vi "svx_Oct_Waterfall Facade.vi"(0 "Data In":T2={"z0"=0.0, "dz"=1.0, "Plots"=[]} {"Plots"."Y" format="%.2f"; "Plots"."X" format="%.2f"}, 2 "Display State In":T5={"X Scale Width %"=50.0, "Y Scale Height %"=50.0, "X-Axis Range"={"Minimum"=0.0, "Maximum"=10.0}, "Y-Axis Range"={"Minimum"=0.0, "Maximum"=10.0}, "Z-Axis Range"={"Minimum"=0.0, "Maximum"=10.0}, "Plot Color"=0, "Frame Color"=61212, "Background Color"=16252785, "Initial AutoScale Y"=TRUE, "AutoScale X"=2, "AutoScale Y"=2, "AutoScale Z"=2, "Plot Transparency"=FALSE, "X-Axis Name"="Frequency", "Y-Axis Name"="Amplitude", "Z-Axis Name"="", "X-Axis Scaling Factor"={"Offset"=0.0, "Multiplier"=1.0}, "Y-Axis Scaling Factor"={"Offset"=0.0, "Multiplier"=1.0}, "Z-Axis Scaling Factor"={"Offset"=0.0, "Multiplier"=1.0}, "X-Scale Visible"=TRUE, "Y-Scale Visible"=TRUE, "Z-Scale Visible"=TRUE, "X-Scale Label Visible"=TRUE, "Y-Scale Label Visible"=TRUE, "Z-Scale Label Visible"=TRUE, "X-Axis Range Scaled"={"Minimum"=0.0, "Maximum"=10.0}, "Y-Axis Range Scaled"={"Minimum"=0.0, "Maximum"=10.0}, "Z-Axis Range Scaled"={"Minimum"=0.0, "Maximum"=10.0}, "Rev Z Order"=FALSE, "X-Scale Format Str"="%#.4g", "Y-Scale Format Str"="%#.4g", "Z-Scale Format Str"="%#.4g", "Decor color"=12369084, "Scale Range Change"=refnum, "out of state queue"=refnum, "property nodes"=refnum}, 3 "Container State":T6) -> (6 "Data Out":T2={"z0"=0.0, "dz"=1.0, "Plots"=[]} {"Plots"."Y" format="%.2f"; "Plots"."X" format="%.2f"}, 7 "Display State Out":T5={"X Scale Width %"=50.0, "Y Scale Height %"=50.0, "X-Axis Range"={"Minimum"=0.0, "Maximum"=10.0}, "Y-Axis Range"={"Minimum"=0.0, "Maximum"=10.0}, "Z-Axis Range"={"Minimum"=0.0, "Maximum"=10.0}, "Plot Color"=0, "Frame Color"=61212, "Background Color"=16252785, "Initial AutoScale Y"=TRUE, "AutoScale X"=2, "AutoScale Y"=2, "AutoScale Z"=2, "Plot Transparency"=FALSE, "X-Axis Name"="Frequency", "Y-Axis Name"="Amplitude", "Z-Axis Name"="", "X-Axis Scaling Factor"={"Offset"=0.0, "Multiplier"=1.0}, "Y-Axis Scaling Factor"={"Offset"=0.0, "Multiplier"=1.0}, "Z-Axis Scaling Factor"={"Offset"=0.0, "Multiplier"=1.0}, "X-Scale Visible"=TRUE, "Y-Scale Visible"=TRUE, "Z-Scale Visible"=TRUE, "X-Scale Label Visible"=TRUE, "Y-Scale Label Visible"=TRUE, "Z-Scale Label Visible"=TRUE, "X-Axis Range Scaled"={"Minimum"=0.0, "Maximum"=10.0}, "Y-Axis Range Scaled"={"Minimum"=0.0, "Maximum"=10.0}, "Z-Axis Range Scaled"={"Minimum"=0.0, "Maximum"=10.0}, "Rev Z Order"=FALSE, "X-Scale Format Str"="%#.4g", "Y-Scale Format Str"="%#.4g", "Z-Scale Format Str"="%#.4g", "Decor color"=12369084, "Scale Range Change"=refnum, "out of state queue"=refnum, "property nodes"=refnum}, 8 "Action":T4)   [LabVIEW 2017, in "SVX Octave Waterfall Graph.xctl"]
uses:
  <vilib>/addons/_XControls/Octave Waterfall Graph/SVX Octave Waterfall Graph.xctl
  <vilib>/addons/_XControls/Octave Waterfall Graph/subVIs/svx_Oct_Waterfall Data.ctl
  <vilib>/_xctls/Container State.ctl
  <vilib>/addons/_XControls/Octave Waterfall Graph/subVIs/svx_Oct_Waterfall State.ctl
  <vilib>/_xctls/Action.ctl
  <vilib>/Utility/miscctls.llb/LVPoint32TypeDef.ctl
  <vilib>/addons/_XControls/Octave Waterfall Graph/subVIs/svx_Oct_Waterfall Execution Tasks.ctl
  <vilib>/Utility/cursorutil.llb/Set Cursor (Icon Pict).vi
  <vilib>/_xctls/XControlSupport.lvlib
panel:
  out "Coords":T1
  out "# Plots Updated":i32
  out "Dec/Cropped":T2={"z0"=0.0, "dz"=1.0, "Plots"=[]} {"Plots"."Y" format="%.2f"; "Plots"."X" format="%.2f"}
  out "Main Graph":T3(graph)
  out "Z Scale Graph":cluster{"f0":dbl, "df":dbl, "magnitude":dbl[]}[](graph)
  out "XY Scale Graph":cluster{"f0":dbl, "df":dbl, "magnitude":dbl[]}[](graph)
  out "background":bool
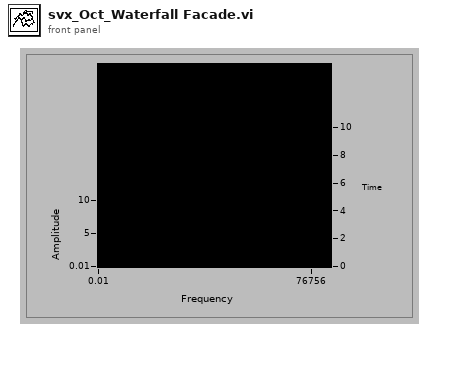
[diagram p1: front panel]
types:
  T1 = typedef "LVPoint32TypeDef.ctl" = cluster{"Horizontal":i32, "Vertical":i32}
  T2 = typedef "SVX Octave Waterfall Graph.xctl/svx_Oct_Waterfall Data.ctl" = cluster{"z0":dbl, "dz":dbl, "Plots":cluster{"X":dbl[], "Y":dbl[]}[]}
  T3 = cluster{"nominal frequencies [Hz]":dbl[], "band power [dB EU]":dbl[]}[]
  T4 = typedef "XControlSupport.lvlib/Action.ctl" = cluster{"Data Changed?":bool, "State Changed?":bool, "Action Name":string}
  T5 = typedef "SVX Octave Waterfall Graph.xctl/svx_Oct_Waterfall State.ctl" = cluster{"X Scale Width %":dbl, "Y Scale Height %":dbl, "X-Axis Range":cluster{"Minimum":dbl, "Maximum":dbl}, "Y-Axis Range":cluster{"Minimum":dbl, "Maximum":dbl}, "Z-Axis Range":cluster{"Minimum":dbl, "Maximum":dbl}, "Plot Color":u32, "Frame Color":u32, "Background Color":u32, "Initial AutoScale Y":bool, "AutoScale X":u8, "AutoScale Y":u8, "AutoScale Z":u8, "Plot Transparency":bool, "X-Axis Name":string, "Y-Axis Name":string, "Z-Axis Name":string, "X-Axis Scaling Factor":cluster{"Offset":dbl, "Multiplier":dbl}, "Y-Axis Scaling Factor":cluster{"Offset":dbl, "Multiplier":dbl}, "Z-Axis Scaling Factor":cluster{"Offset":dbl, "Multiplier":dbl}, "X-Scale Visible":bool, "Y-Scale Visible":bool, "Z-Scale Visible":bool, "X-Scale Label Visible":bool, "Y-Scale Label Visible":bool, "Z-Scale Label Visible":bool, "X-Axis Range Scaled":cluster{"Minimum":dbl, "Maximum":dbl}, "Y-Axis Range Scaled":cluster{"Minimum":dbl, "Maximum":dbl}, "Z-Axis Range Scaled":cluster{"Minimum":dbl, "Maximum":dbl}, "Rev Z Order":bool, "X-Scale Format Str":string, "Y-Scale Format Str":string, "Z-Scale Format Str":string, "Decor color":u32, "Scale Range Change":refnum<user-event>, "out of state queue":refnum<queue>, "property nodes":refnum<queue>}
  T6 = typedef "XControlSupport.lvlib/Container State.ctl" = cluster{"Indicator?":bool, "Run Mode?":bool, " Refnum":refnum<vi>}
  T7 = cluster{"Grabbing?":bool, "Coords":T1, "Time":u32}
  T8 = typedef "SVX Octave Waterfall Graph.xctl/svx_Oct_Waterfall Execution Tasks.ctl" = enum16{"[Data] Default", "[Data] Update Graph", "[Pane] Calculate Size from Coord Change", "[Pane] Calculate Size from Display State", "[Plot] Redraw Frame", "[Plot] Update Plot Color", "[Scale] Autoscale or Crop X, Y, Z", "[Scale] Resize Scales", "[Scale] Align Scale Labels", "[Plot] Initialize Plot", "[Scale] X Scale", "[Scale] Y Scale", "[Scale] Z Scale", "[Scale] Multiplier/Offset", "[Scale] Name", "[Scale] Visible", "[Scale] Label Visible", "[Scale] Format"}
  T9 = cluster{"use queue?":bool, "X-Axis Range":cluster{"Minimum":dbl, "Maximum":dbl}, "Y-Axis Range":cluster{"Minimum":dbl, "Maximum":dbl}, "Z-Axis Range":cluster{"Minimum":dbl, "Maximum":dbl}, "X-Axis Range Scaled":cluster{"Minimum":dbl, "Maximum":dbl}, "Y-Axis Range Scaled":cluster{"Minimum":dbl, "Maximum":dbl}, "Z-Axis Range Scaled":cluster{"Minimum":dbl, "Maximum":dbl}, "AutoScale X":u8, "AutoScale Y":u8, "AutoScale Z":u8, "background":refnum<vi>}
  T10 = cluster{"Scaled.Minimum":dbl, "Scaled.Maximum":dbl, "Kind":enum16{"X-Scale", "Y-Scale", "Z-Scale"}}
  T11 = cluster{"Range.Minimum":dbl, "Range.Maximum":dbl, "Kind":enum16{"X-Scale", "Y-Scale", "Z-Scale"}}
  T12 = typedef "LVRectTypeDef.ctl" = cluster{"Left":i16, "Top":i16, "Right":i16, "Bottom":i16}
  T13 = typedef "LVPositionTypeDef.ctl" = cluster{"Left":i32, "Top":i32}
  T14 = cluster{"Shift":bool, "Ctrl":bool, "Alt":bool, "Cmd":bool, "Opt":bool}
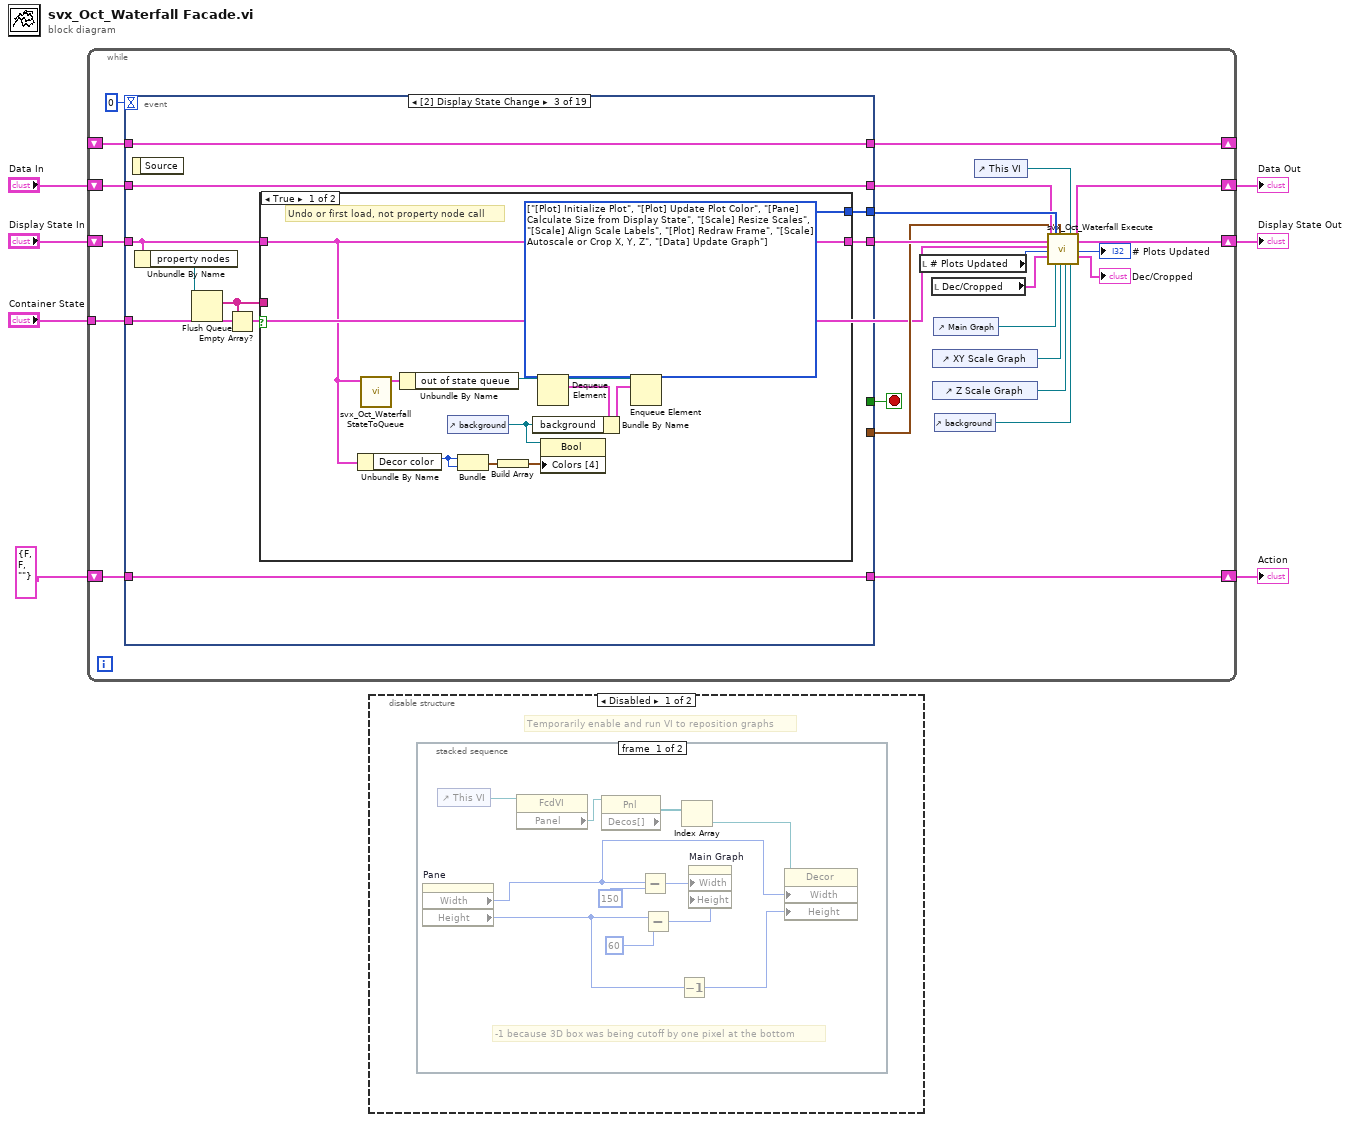
[diagram p0: block diagram]
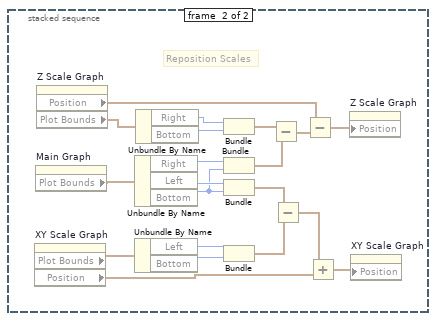
[diagram p2: hidden frame]
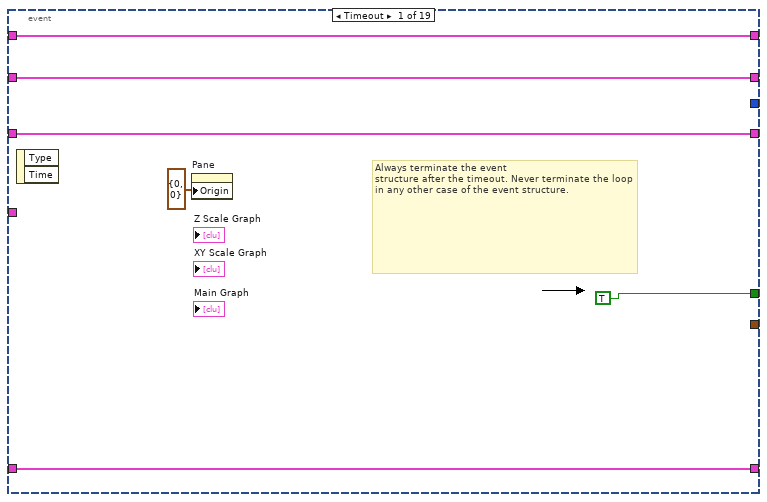
[diagram p4: hidden frame]
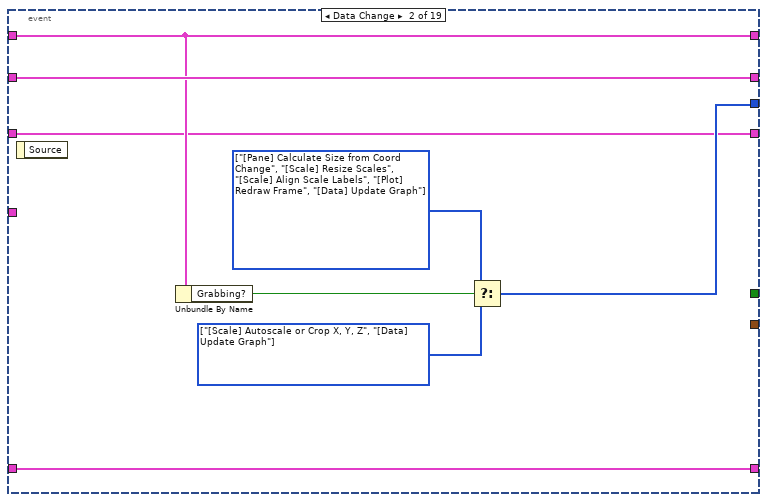
[diagram p5: hidden frame]
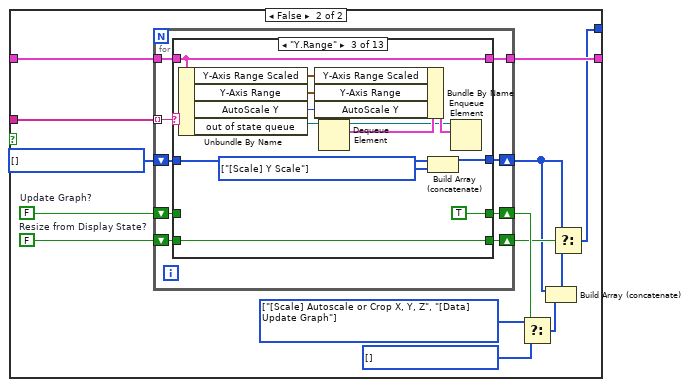
[diagram p6: hidden frame]
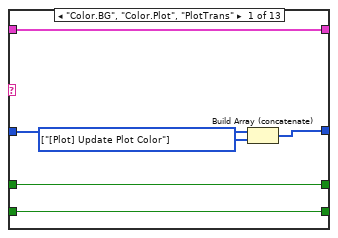
[diagram p7: hidden frame]
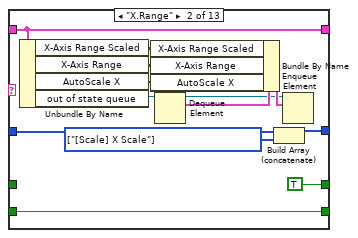
[diagram p8: hidden frame]
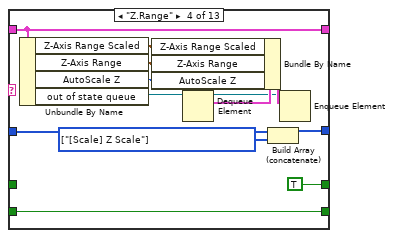
[diagram p9: hidden frame]
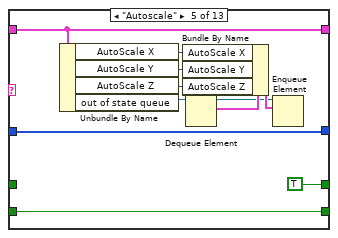
[diagram p10: hidden frame]
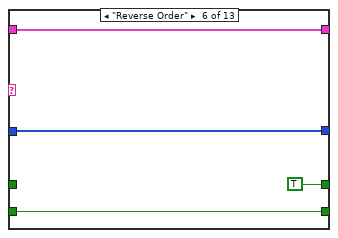
[diagram p11: hidden frame]
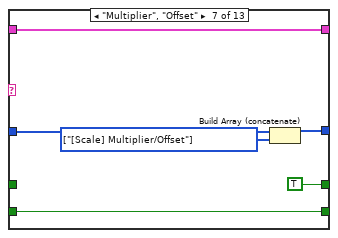
[diagram p12: hidden frame]
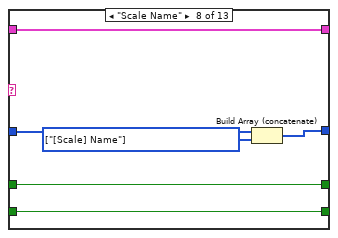
[diagram p13: hidden frame]
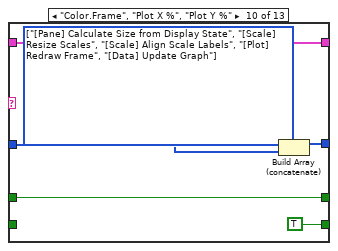
[diagram p15: hidden frame]
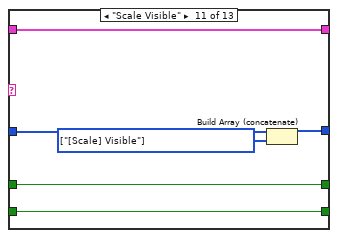
[diagram p16: hidden frame]
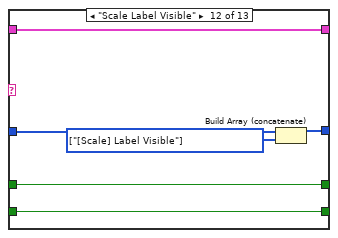
[diagram p17: hidden frame]
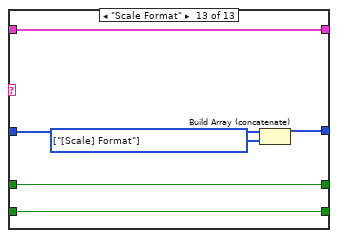
[diagram p18: hidden frame]
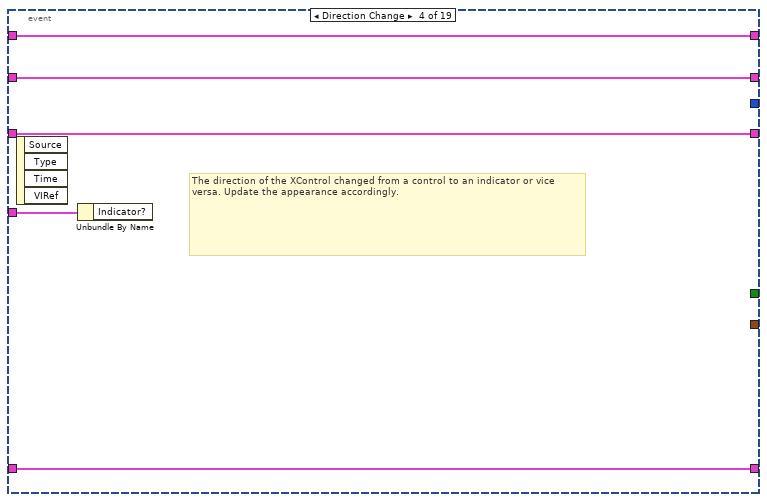
[diagram p19: hidden frame]
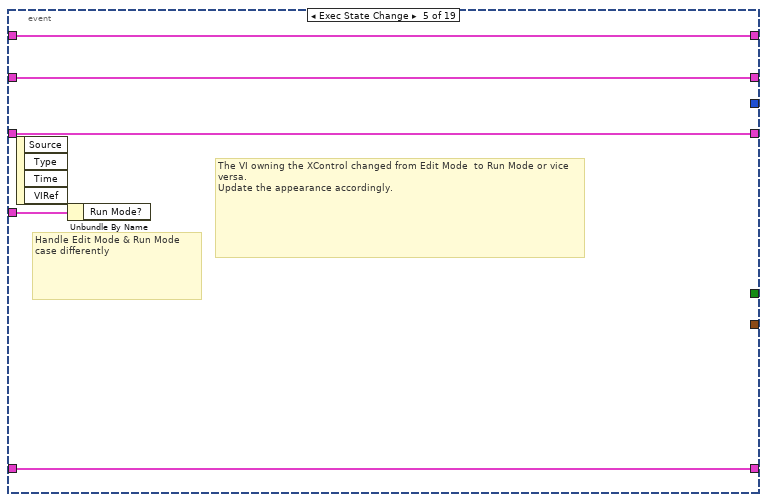
[diagram p20: hidden frame]
diagram:
  n1 = while {
    shift-right: [w12] -> w4
    shift-left: "Display State In" -> [w31]
    tunnel: "Container State" -> [w17]
    shift-right: [w20] -> w7
    shift-left: "Data In" -> [w28]
    shift-right: [w24] -> w2
    shift-left: T4 {"Data Changed?"=FALSE, "State Changed?"=FALSE, "Action Name"=""} ("Action") -> [w27]
    shift-right: [w25] -> _
    shift-left: _ -> [w26]
    stop <- w30 stop-if-true
    n2 = event shown="[2] Display State Change" {
      selector: _ -> [_ _ _ _ _ _ _ _ _ _ _ _ _ _ _ _ _ _ _]
      dyn-events: _ -> [_ _ _ _ _ _ _ _ _ _ _ _ _ _ _ _ _ _ _]
      timeout: 0 -> [_ _ _ _ _ _ _ _ _ _ _ _ _ _ _ _ _ _ _]
      tunnel: w31 -> [w32 w38 w51 w192 w197 w200 w227 w255 w290 w308 w315 w325 w385 w405 w447 w461 w479 w628 w654]
      tunnel: [w32 w38 w52 w192 w197 w199 w227 w255 w290 w308 w314 w325 w386 w405 w447 w461 w478 w628 w654] -> w22
      tunnel: [TRUE _ _ _ _ _ _ _ _ _ _ _ _ _ _ _ _ _ _] -> w30
      tunnel: w17 -> [_ _ _ w193 w198 w206 _ w254 w285 _ _ _ _ _ w448 w460 w474 _ _]
      tunnel: w28 -> [w36 w45 w53 w191 w196 w215 w230 w259 w289 w310 w321 w336 w399 w407 w454 w463 w475 w632 w655]
      tunnel: [w36 w45 w53 w191 w196 w215 w230 w259 w289 w310 w321 w336 w399 w407 w454 w463 w475 w631 w655] -> w21
      tunnel: [w33 w42 w47 w190 w195 w203 w226 w252 w283 w307 w312 w338 w400 w406 w455 w464 w476 w629 w648] -> w24
      tunnel: w27 -> [w33 w42 w47 w190 w195 w204 w226 w253 w284 w307 w313 w339 w401 w406 w455 w464 w477 w630 w648]
      tunnel: [w34 w44 w54 w189 w194 w214 w240 w262 w288 w309 w320 w341 w403 w409 w453 w462 w480 w635 w656] -> w25
      tunnel: w26 -> [w34 w44 w54 w189 w194 _ w239 w261 w287 w309 w320 w341 w403 w409 w453 w462 w480 w635 w656]
      tunnel: [_ _ _ _ _ _ w228 w256 _ _ _ _ _ _ _ _ _ _ _] -> w18
      tunnel: [_ w39 w46 _ _ _ w225 w251 w282 _ _ w328 w370 w404 _ _ w473 w627 _] -> w23
      event Timeout {
        # "Always terminate the event\nstructure after the timeout. Never terminate the loop in any other case of the event structure."
        n3 = event-data() -> ()  [unwired: 1 in, 2 out]
        n4 = property on="Pane" class="Pane"("Origin"=cluster{"Horizontal":i16, "Vertical":i16} {"Horizontal"=0, "Vertical"=0}) -> ()  [unwired: 2 in, 2 out]
      }
      event Data Change {
        w40 = T8[] [enum."[Scale] Autoscale or Crop X, Y, Z", enum."[Data] Update Graph"] items=["[Data] Default", "[Data] Update Graph", "[Pane] Calculate Size from Coord Change", "[Pane] Calculate Size from Display State", "[Plot] Redraw Frame", "[Plot] Update Plot Color", "[Scale] Autoscale or Crop X, Y, Z", "[Scale] Resize Scales", "[Scale] Align Scale Labels", "[Plot] Initialize Plot", "[Scale] X Scale", "[Scale] Y Scale", "[Scale] Z Scale", "[Scale] Multiplier/Offset", "[Scale] Name", "[Scale] Visible", "[Scale] Label Visible", "[Scale] Format"] ("element")
        w41 = T8[] [enum."[Pane] Calculate Size from Coord Change", enum."[Scale] Resize Scales", enum."[Scale] Align Scale Labels", enum."[Plot] Redraw Frame", enum."[Data] Update Graph"] items=["[Data] Default", "[Data] Update Graph", "[Pane] Calculate Size from Coord Change", "[Pane] Calculate Size from Display State", "[Plot] Redraw Frame", "[Plot] Update Plot Color", "[Scale] Autoscale or Crop X, Y, Z", "[Scale] Resize Scales", "[Scale] Align Scale Labels", "[Plot] Initialize Plot", "[Scale] X Scale", "[Scale] Y Scale", "[Scale] Z Scale", "[Scale] Multiplier/Offset", "[Scale] Name", "[Scale] Visible", "[Scale] Label Visible", "[Scale] Format"] ("element")
        n5 = event-data() -> ()  [unwired: 1 in, 1 out]
        n6 = Unbundle By Name(w44) -> ("Grabbing?"=w43:bool)
        n7 = Select(t=w41, s=w43, f=w40) -> (s? t:f=w39:T8[])
      }
      event Display State Change {
        n8 = event-data() -> ()  [unwired: 1 in, 1 out]
        n9 = Unbundle By Name(w51) -> ("property nodes"=w50:refnum<queue>)
        n10 = Flush Queue(queue=w50) -> (remaining elements=w48:string[])  [unwired: 1 in, 2 out]
        n11 = Empty Array?(array=w48) -> (empty?=w49:bool)
        n12 = case shown="True" w49 {
          tunnel: [w61 w79] -> w52
          tunnel: w51 -> [w61 w78]
          tunnel: [w60 w66] -> w46
          tunnel: w48 -> [_ w77]
          frame True {
            w60 = T8[] [enum."[Plot] Initialize Plot", enum."[Plot] Update Plot Color", enum."[Pane] Calculate Size from Display State", enum."[Scale] Resize Scales", enum."[Scale] Align Scale Labels", enum."[Plot] Redraw Frame", enum."[Scale] Autoscale or Crop X, Y, Z", enum."[Data] Update Graph"] items=["[Data] Default", "[Data] Update Graph", "[Pane] Calculate Size from Coord Change", "[Pane] Calculate Size from Display State", "[Plot] Redraw Frame", "[Plot] Update Plot Color", "[Scale] Autoscale or Crop X, Y, Z", "[Scale] Resize Scales", "[Scale] Align Scale Labels", "[Plot] Initialize Plot", "[Scale] X Scale", "[Scale] Y Scale", "[Scale] Z Scale", "[Scale] Multiplier/Offset", "[Scale] Name", "[Scale] Visible", "[Scale] Label Visible", "[Scale] Format"]
            # "Undo or first load, not property node call"
            n13 = Unbundle By Name(w61) -> ("Decor color"=w57:u32)
            n14 = call <vilib>:"svx_Oct_Waterfall StateToQueue.vi"("State In"=w61) -> ("State Out"=w65:T5)  [unwired: 10 in]
            n15 = Unbundle By Name(w65) -> ("out of state queue"=w62:refnum<queue>)
            n16 = control-ref of="background"() -> (w58:refnum<vi>)
            n17 = Bundle("Decor color"=w57, "Decor color"=w57) -> (w55:cluster{"Decor color":u32, "Decor color":u32})  [unwired: 1 in]
            n18 = Build Array(w55) -> (w56:cluster{"Decor color":u32, "Decor color":u32}[])
            n19 = Dequeue Element(queue=w62) -> (queue out=w59:refnum<queue>, element=w63:T9)  [unwired: 2 in, 2 out]
            n20 = Bundle By Name(cluster=w63, "background"=w58) -> (w64:T9)
            n21 = property on="Property Node" class="Bool"(reference=w58, "Colors [4]"=w56) -> ()  [unwired: 1 in, 2 out]
            n22 = Enqueue Element(queue=w59, element=w64) -> ()  [unwired: 2 in, 3 out]
          }
          frame False {
            w71 = T8[] [] items=["[Data] Default", "[Data] Update Graph", "[Pane] Calculate Size from Coord Change", "[Pane] Calculate Size from Display State", "[Plot] Redraw Frame", "[Plot] Update Plot Color", "[Scale] Autoscale or Crop X, Y, Z", "[Scale] Resize Scales", "[Scale] Align Scale Labels", "[Plot] Initialize Plot", "[Scale] X Scale", "[Scale] Y Scale", "[Scale] Z Scale", "[Scale] Multiplier/Offset", "[Scale] Name", "[Scale] Visible", "[Scale] Label Visible", "[Scale] Format"]
            w72 = T8[] [enum."[Scale] Autoscale or Crop X, Y, Z", enum."[Data] Update Graph"] items=["[Data] Default", "[Data] Update Graph", "[Pane] Calculate Size from Coord Change", "[Pane] Calculate Size from Display State", "[Plot] Redraw Frame", "[Plot] Update Plot Color", "[Scale] Autoscale or Crop X, Y, Z", "[Scale] Resize Scales", "[Scale] Align Scale Labels", "[Plot] Initialize Plot", "[Scale] X Scale", "[Scale] Y Scale", "[Scale] Z Scale", "[Scale] Multiplier/Offset", "[Scale] Name", "[Scale] Visible", "[Scale] Label Visible", "[Scale] Format"]
            w76 = T8[] [] items=["[Data] Default", "[Data] Update Graph", "[Pane] Calculate Size from Coord Change", "[Pane] Calculate Size from Display State", "[Plot] Redraw Frame", "[Plot] Update Plot Color", "[Scale] Autoscale or Crop X, Y, Z", "[Scale] Resize Scales", "[Scale] Align Scale Labels", "[Plot] Initialize Plot", "[Scale] X Scale", "[Scale] Y Scale", "[Scale] Z Scale", "[Scale] Multiplier/Offset", "[Scale] Name", "[Scale] Visible", "[Scale] Label Visible", "[Scale] Format"]
            w74 = FALSE  # Resize from Display State?
            w75 = FALSE  # Update Graph?
            n23 = for {
              tunnel: [w88] -> w79
              tunnel: w77 -> [w87] mode=indexing
              tunnel: w78 -> [w86]
              shift-right: [w84] -> w68
              shift-left: w76 -> [w85]
              shift-right: [w83] -> w73
              shift-left: w75 -> [w82]
              shift-right: [w80] -> w70
              shift-left: w74 -> [w81]
              n24 = case shown="\"Y.Range\"" w87 {
                tunnel: [w94 w96 w110 w122 w135 w148 w154 w160 w164 w170 w176 w182 w188] -> w88
                tunnel: w86 -> [w94 w96 w110 w122 w135 w148 w154 w160 w164 w170 w176 w182 w188]
                tunnel: w85 -> [w93 w104 w117 w130 w144 w147 w150 w158 w163 w167 w172 w179 w185]
                tunnel: [w91 w105 w118 w131 w144 w147 w151 w157 w163 w168 w173 w180 w186] -> w84
                tunnel: [w90 TRUE ("Update Graph?") TRUE ("Update Graph?") TRUE ("Update Graph?") TRUE ("Update Graph?") TRUE ("Update Graph?") TRUE ("Update Graph?") w156 w162 w169 w175 w178 w184] -> w83
                tunnel: w82 -> [w90 _ _ _ _ _ _ w156 w162 w169 w175 w178 w184]
                tunnel: w81 -> [w89 w95 w109 w121 w134 w145 w149 w155 w161 _ w171 w177 w183]
                tunnel: [w89 w95 w109 w121 w134 w145 w149 w155 w161 TRUE ("Resize from Display State?") w171 w177 w183] -> w80
                frame "Color.BG", "Color.Plot", "PlotTrans" {
                  w92 = T8[] [enum."[Plot] Update Plot Color"] items=["[Data] Default", "[Data] Update Graph", "[Pane] Calculate Size from Coord Change", "[Pane] Calculate Size from Display State", "[Plot] Redraw Frame", "[Plot] Update Plot Color", "[Scale] Autoscale or Crop X, Y, Z", "[Scale] Resize Scales", "[Scale] Align Scale Labels", "[Plot] Initialize Plot", "[Scale] X Scale", "[Scale] Y Scale", "[Scale] Z Scale", "[Scale] Multiplier/Offset", "[Scale] Name", "[Scale] Visible", "[Scale] Label Visible", "[Scale] Format"] ("element")
                  n25 = Build Array (concatenate)(w93, w92) -> (w91:T8[])
                }
                frame "X.Range" {
                  w106 = T8[] [enum."[Scale] X Scale"] items=["[Data] Default", "[Data] Update Graph", "[Pane] Calculate Size from Coord Change", "[Pane] Calculate Size from Display State", "[Plot] Redraw Frame", "[Plot] Update Plot Color", "[Scale] Autoscale or Crop X, Y, Z", "[Scale] Resize Scales", "[Scale] Align Scale Labels", "[Plot] Initialize Plot", "[Scale] X Scale", "[Scale] Y Scale", "[Scale] Z Scale", "[Scale] Multiplier/Offset", "[Scale] Name", "[Scale] Visible", "[Scale] Label Visible", "[Scale] Format"] ("element")
                  n26 = Unbundle By Name(w96) -> ("X-Axis Range Scaled"=w101:cluster{"Minimum":dbl, "Maximum":dbl}, "X-Axis Range"=w103:cluster{"Minimum":dbl, "Maximum":dbl}, "AutoScale X"=w102:u8, "out of state queue"=w97:refnum<queue>)
                  n27 = Dequeue Element(queue=w97) -> (queue out=w98:refnum<queue>, element=w99:T9)  [unwired: 2 in, 2 out]
                  n28 = Bundle By Name(cluster=w99, "X-Axis Range Scaled"=w101, "X-Axis Range"=w103, "AutoScale X"=w102) -> (w100:T9)
                  n29 = Build Array (concatenate)(w104, w106) -> (w105:T8[])
                  n30 = Enqueue Element(queue=w98, element=w100) -> ()  [unwired: 2 in, 3 out]
                }
                frame "Y.Range" {
                  w119 = T8[] [enum."[Scale] Y Scale"] items=["[Data] Default", "[Data] Update Graph", "[Pane] Calculate Size from Coord Change", "[Pane] Calculate Size from Display State", "[Plot] Redraw Frame", "[Plot] Update Plot Color", "[Scale] Autoscale or Crop X, Y, Z", "[Scale] Resize Scales", "[Scale] Align Scale Labels", "[Plot] Initialize Plot", "[Scale] X Scale", "[Scale] Y Scale", "[Scale] Z Scale", "[Scale] Multiplier/Offset", "[Scale] Name", "[Scale] Visible", "[Scale] Label Visible", "[Scale] Format"] ("element")
                  n31 = Unbundle By Name(w110) -> ("Y-Axis Range Scaled"=w108:cluster{"Minimum":dbl, "Maximum":dbl}, "Y-Axis Range"=w115:cluster{"Minimum":dbl, "Maximum":dbl}, "AutoScale Y"=w116:u8, "out of state queue"=w112:refnum<queue>)
                  n32 = Dequeue Element(queue=w112) -> (queue out=w111:refnum<queue>, element=w113:T9)  [unwired: 2 in, 2 out]
                  n33 = Bundle By Name(cluster=w113, "Y-Axis Range Scaled"=w108, "Y-Axis Range"=w115, "AutoScale Y"=w116) -> (w114:T9)
                  n34 = Build Array (concatenate)(w117, w119) -> (w118:T8[])
                  n35 = Enqueue Element(queue=w111, element=w114) -> ()  [unwired: 2 in, 3 out]
                }
                frame "Z.Range" {
                  w132 = T8[] [enum."[Scale] Z Scale"] items=["[Data] Default", "[Data] Update Graph", "[Pane] Calculate Size from Coord Change", "[Pane] Calculate Size from Display State", "[Plot] Redraw Frame", "[Plot] Update Plot Color", "[Scale] Autoscale or Crop X, Y, Z", "[Scale] Resize Scales", "[Scale] Align Scale Labels", "[Plot] Initialize Plot", "[Scale] X Scale", "[Scale] Y Scale", "[Scale] Z Scale", "[Scale] Multiplier/Offset", "[Scale] Name", "[Scale] Visible", "[Scale] Label Visible", "[Scale] Format"] ("element")
                  n36 = Unbundle By Name(w122) -> ("Z-Axis Range Scaled"=w126:cluster{"Minimum":dbl, "Maximum":dbl}, "Z-Axis Range"=w127:cluster{"Minimum":dbl, "Maximum":dbl}, "AutoScale Z"=w125:u8, "out of state queue"=w124:refnum<queue>)
                  n37 = Dequeue Element(queue=w124) -> (queue out=w123:refnum<queue>, element=w128:T9)  [unwired: 2 in, 2 out]
                  n38 = Bundle By Name(cluster=w128, "Z-Axis Range Scaled"=w126, "Z-Axis Range"=w127, "AutoScale Z"=w125) -> (w129:T9)
                  n39 = Build Array (concatenate)(w130, w132) -> (w131:T8[])
                  n40 = Enqueue Element(queue=w123, element=w129) -> ()  [unwired: 2 in, 3 out]
                }
                frame "Autoscale" {
                  n41 = Unbundle By Name(w135) -> ("AutoScale X"=w140:u8, "AutoScale Y"=w141:u8, "AutoScale Z"=w142:u8, "out of state queue"=w137:refnum<queue>)
                  n42 = Dequeue Element(queue=w137) -> (queue out=w136:refnum<queue>, element=w138:T9)  [unwired: 2 in, 2 out]
                  n43 = Bundle By Name(cluster=w138, "AutoScale X"=w140, "AutoScale Y"=w141, "AutoScale Z"=w142) -> (w139:T9)
                  n44 = Enqueue Element(queue=w136, element=w139) -> ()  [unwired: 2 in, 3 out]
                }
                frame "Reverse Order" {
                }
                frame "Multiplier", "Offset" {
                  w152 = T8[] [enum."[Scale] Multiplier/Offset"] items=["[Data] Default", "[Data] Update Graph", "[Pane] Calculate Size from Coord Change", "[Pane] Calculate Size from Display State", "[Plot] Redraw Frame", "[Plot] Update Plot Color", "[Scale] Autoscale or Crop X, Y, Z", "[Scale] Resize Scales", "[Scale] Align Scale Labels", "[Plot] Initialize Plot", "[Scale] X Scale", "[Scale] Y Scale", "[Scale] Z Scale", "[Scale] Multiplier/Offset", "[Scale] Name", "[Scale] Visible", "[Scale] Label Visible", "[Scale] Format"] ("element")
                  n45 = Build Array (concatenate)(w150, w152) -> (w151:T8[])
                }
                frame "Scale Name" {
                  w159 = T8[] [enum."[Scale] Name"] items=["[Data] Default", "[Data] Update Graph", "[Pane] Calculate Size from Coord Change", "[Pane] Calculate Size from Display State", "[Plot] Redraw Frame", "[Plot] Update Plot Color", "[Scale] Autoscale or Crop X, Y, Z", "[Scale] Resize Scales", "[Scale] Align Scale Labels", "[Plot] Initialize Plot", "[Scale] X Scale", "[Scale] Y Scale", "[Scale] Z Scale", "[Scale] Multiplier/Offset", "[Scale] Name", "[Scale] Visible", "[Scale] Label Visible", "[Scale] Format"] ("element")
                  n46 = Build Array (concatenate)(w158, w159) -> (w157:T8[])
                }
                frame Default {
                }
                frame "Color.Frame", "Plot X %", "Plot Y %" {
                  w166 = T8[] [enum."[Pane] Calculate Size from Display State", enum."[Scale] Resize Scales", enum."[Scale] Align Scale Labels", enum."[Plot] Redraw Frame", enum."[Data] Update Graph"] items=["[Data] Default", "[Data] Update Graph", "[Pane] Calculate Size from Coord Change", "[Pane] Calculate Size from Display State", "[Plot] Redraw Frame", "[Plot] Update Plot Color", "[Scale] Autoscale or Crop X, Y, Z", "[Scale] Resize Scales", "[Scale] Align Scale Labels", "[Plot] Initialize Plot", "[Scale] X Scale", "[Scale] Y Scale", "[Scale] Z Scale", "[Scale] Multiplier/Offset", "[Scale] Name", "[Scale] Visible", "[Scale] Label Visible", "[Scale] Format"]
                  n47 = Build Array (concatenate)(w167, w166) -> (w168:T8[])
                }
                frame "Scale Visible" {
                  w174 = T8[] [enum."[Scale] Visible"] items=["[Data] Default", "[Data] Update Graph", "[Pane] Calculate Size from Coord Change", "[Pane] Calculate Size from Display State", "[Plot] Redraw Frame", "[Plot] Update Plot Color", "[Scale] Autoscale or Crop X, Y, Z", "[Scale] Resize Scales", "[Scale] Align Scale Labels", "[Plot] Initialize Plot", "[Scale] X Scale", "[Scale] Y Scale", "[Scale] Z Scale", "[Scale] Multiplier/Offset", "[Scale] Name", "[Scale] Visible", "[Scale] Label Visible", "[Scale] Format"] ("element")
                  n48 = Build Array (concatenate)(w172, w174) -> (w173:T8[])
                }
                frame "Scale Label Visible" {
                  w181 = T8[] [enum."[Scale] Label Visible"] items=["[Data] Default", "[Data] Update Graph", "[Pane] Calculate Size from Coord Change", "[Pane] Calculate Size from Display State", "[Plot] Redraw Frame", "[Plot] Update Plot Color", "[Scale] Autoscale or Crop X, Y, Z", "[Scale] Resize Scales", "[Scale] Align Scale Labels", "[Plot] Initialize Plot", "[Scale] X Scale", "[Scale] Y Scale", "[Scale] Z Scale", "[Scale] Multiplier/Offset", "[Scale] Name", "[Scale] Visible", "[Scale] Label Visible", "[Scale] Format"] ("element")
                  n49 = Build Array (concatenate)(w179, w181) -> (w180:T8[])
                }
                frame "Scale Format" {
                  w187 = T8[] [enum."[Scale] Format"] items=["[Data] Default", "[Data] Update Graph", "[Pane] Calculate Size from Coord Change", "[Pane] Calculate Size from Display State", "[Plot] Redraw Frame", "[Plot] Update Plot Color", "[Scale] Autoscale or Crop X, Y, Z", "[Scale] Resize Scales", "[Scale] Align Scale Labels", "[Plot] Initialize Plot", "[Scale] X Scale", "[Scale] Y Scale", "[Scale] Z Scale", "[Scale] Multiplier/Offset", "[Scale] Name", "[Scale] Visible", "[Scale] Label Visible", "[Scale] Format"] ("element")
                  n50 = Build Array (concatenate)(w185, w187) -> (w186:T8[])
                }
              }
            }
            n51 = Select(t=w72, s=w73, f=w71) -> (s? t:f=w69:T8[])
            n52 = Build Array (concatenate)(w68, w69) -> (w67:T8[])
            n53 = Select(t=w68, s=w70, f=w67) -> (s? t:f=w66:T8[])
          }
        }
      }
      event Direction Change {
        # "The direction of the XControl changed from a control to an indicator or vice versa. Update the appearance accordingly."
        n54 = event-data() -> ()  [unwired: 1 in, 4 out]
        n55 = Unbundle By Name(w193) -> ()  [unwired: 1 out]
      }
      event Exec State Change {
        # "The VI owning the XControl changed from Edit Mode  to Run Mode or vice versa.\nUpdate the appearance accordingly."
        # "Handle Edit Mode & Run Mode\ncase differently"
        n56 = event-data() -> ()  [unwired: 1 in, 4 out]
        n57 = Unbundle By Name(w198) -> ()  [unwired: 1 out]
      }
      event "Main Graph": Mouse Down? {
        n58 = event-data() -> ("Coords"=w213:T1, "PlatMods.Ctrl"=w209:bool, "Button"=w211:u16)  [unwired: 1 in]
        n59 = Unbundle By Name(w200) -> ("Background Color"=w205:u32)
        n60 = Equal?(x=w211, y=u16 1) -> (x = y?=w208:bool)
        n61 = property on="Main Graph" class="XYGraph (strict)"() -> ("BG Color"=w201:u32)  [unwired: 2 in, 2 out]
        n62 = And(x=w209, y=w208) -> (x .and. y?=w207:bool)
        n63 = Not Equal?(x=w201, y=w205) -> (x != y?=w202:bool)
        n64 = case shown="True" w207 {
          tunnel: [w216 w224] -> w214
          tunnel: w213 -> [_ w222]
          tunnel: T7 {"Grabbing?"=FALSE, "Coords"={"Horizontal"=0, "Vertical"=0}, "Time"=0} -> [w216 w221]
          tunnel: w206 -> [_ w220]
          frame False {
          }
          frame True {
            n65 = Unbundle By Name(w220) -> ("Refnum"=w219:refnum<vi>)
            n66 = property class="Ctl"(reference=w219) -> ("OwningVI"=w218:refnum<vi>)  [unwired: 1 in, 2 out]
            n67 = Bundle By Name(cluster=w221, "Grabbing?"=TRUE, "Coords"=w222) -> (w224:T7)
            n68 = call-poly <vilib>:"Set Cursor.vi"("VI reference (current VI)"=w218, "icon"=u16 11) -> ()  [unwired: 8 in, 2 out]
          }
        }
        n69 = Bundle By Name(cluster=w204, "State Changed?"=w202) -> (w203:T4)
        n70 = Bundle By Name(cluster=w200, "Background Color"=w201) -> (w199:T5)
        n71 = event-data() -> ()  [unwired: 2 in, 1 out]
      }
      event "Main Graph": Mouse Move {
        # "Time delay so \nwe don't execute\nevery event"
        n72 = event-data() -> ("Time"=w231:u32, "Coords"=w232:T1)  [unwired: 1 in]
        n73 = Unbundle By Name(w239) -> ("Coords"=w233:T1, "Grabbing?"=w236:bool, "Time"=w238:u32)
        n74 = Subtract(x=w231, y=w238) -> (x-y=w237:u32)
        n75 = Greater Or Equal?(x=w237, y=u32 50 ("delay")) -> (x >= y?=w235:bool)
        n76 = And(x=w236, y=w235) -> (x .and. y?=w234:bool)
        n77 = case shown="True" w234 {
          tunnel: [w243 w250] -> w240
          tunnel: w239 -> [w243 w249]
          tunnel: w233 -> [_ w248]
          tunnel: w232 -> [_ w246]
          tunnel: w231 -> [_ w247]
          tunnel: [cluster{"Horizontal":i32, "Vertical":i32} {"Horizontal"=0, "Vertical"=0} w245] -> w228
          tunnel: [w241 w244] -> w225
          frame False {
            w241 = T8[] [] items=["[Data] Default", "[Data] Update Graph", "[Pane] Calculate Size from Coord Change", "[Pane] Calculate Size from Display State", "[Plot] Redraw Frame", "[Plot] Update Plot Color", "[Scale] Autoscale or Crop X, Y, Z", "[Scale] Resize Scales", "[Scale] Align Scale Labels", "[Plot] Initialize Plot", "[Scale] X Scale", "[Scale] Y Scale", "[Scale] Z Scale", "[Scale] Multiplier/Offset", "[Scale] Name", "[Scale] Visible", "[Scale] Label Visible", "[Scale] Format"] ("element")
          }
          frame True {
            w244 = T8[] [enum."[Pane] Calculate Size from Coord Change", enum."[Scale] Resize Scales", enum."[Scale] Align Scale Labels", enum."[Plot] Redraw Frame", enum."[Data] Update Graph"] items=["[Data] Default", "[Data] Update Graph", "[Pane] Calculate Size from Coord Change", "[Pane] Calculate Size from Display State", "[Plot] Redraw Frame", "[Plot] Update Plot Color", "[Scale] Autoscale or Crop X, Y, Z", "[Scale] Resize Scales", "[Scale] Align Scale Labels", "[Plot] Initialize Plot", "[Scale] X Scale", "[Scale] Y Scale", "[Scale] Z Scale", "[Scale] Multiplier/Offset", "[Scale] Name", "[Scale] Visible", "[Scale] Label Visible", "[Scale] Format"] ("element")
            n78 = Subtract(x=w246, y=w248) -> (x-y=w245:T1)
            n79 = Bundle By Name(cluster=w249, "Time"=w247, "Coords"=w246) -> (w250:T7)
          }
        }
      }
      event "Main Graph": Mouse Up {
        n80 = event-data() -> ("Coords"=w258:T1)  [unwired: 1 in]
        n81 = Unbundle By Name(w261) -> ("Grabbing?"=w260:bool, "Coords"=w257:T1)
        n82 = case shown="True" w260 {
          tunnel: [w266 w278] -> w262
          tunnel: w261 -> [w266 w279]
          tunnel: w258 -> [_ w281]
          tunnel: w257 -> [_ w280]
          tunnel: [cluster{"Horizontal":i32, "Vertical":i32} {"Horizontal"=0, "Vertical"=0} w276] -> w256
          tunnel: w254 -> [_ w272]
          tunnel: w253 -> [w264 w271]
          tunnel: [w264 w270] -> w252
          tunnel: [w263 w267] -> w251
          frame False {
            w263 = T8[] [] items=["[Data] Default", "[Data] Update Graph", "[Pane] Calculate Size from Coord Change", "[Pane] Calculate Size from Display State", "[Plot] Redraw Frame", "[Plot] Update Plot Color", "[Scale] Autoscale or Crop X, Y, Z", "[Scale] Resize Scales", "[Scale] Align Scale Labels", "[Plot] Initialize Plot", "[Scale] X Scale", "[Scale] Y Scale", "[Scale] Z Scale", "[Scale] Multiplier/Offset", "[Scale] Name", "[Scale] Visible", "[Scale] Label Visible", "[Scale] Format"] ("element")
          }
          frame True {
            w267 = T8[] [enum."[Pane] Calculate Size from Coord Change", enum."[Scale] Resize Scales", enum."[Scale] Align Scale Labels", enum."[Plot] Redraw Frame", enum."[Data] Update Graph"] items=["[Data] Default", "[Data] Update Graph", "[Pane] Calculate Size from Coord Change", "[Pane] Calculate Size from Display State", "[Plot] Redraw Frame", "[Plot] Update Plot Color", "[Scale] Autoscale or Crop X, Y, Z", "[Scale] Resize Scales", "[Scale] Align Scale Labels", "[Plot] Initialize Plot", "[Scale] X Scale", "[Scale] Y Scale", "[Scale] Z Scale", "[Scale] Multiplier/Offset", "[Scale] Name", "[Scale] Visible", "[Scale] Label Visible", "[Scale] Format"] ("element")
            n83 = Unbundle By Name(w272) -> ("Refnum"=w275:refnum<vi>)
            n84 = Subtract(x=w281, y=w280) -> (x-y=w276:T1)
            n85 = property class="Ctl"(reference=w275) -> ("OwningVI"=w274:refnum<vi>)  [unwired: 1 in, 2 out]
            n86 = call-poly <vilib>:"Set Cursor.vi"("VI reference (current VI)"=w274, "icon"=u16 0) -> ()  [unwired: 8 in, 2 out]
            n87 = Bundle By Name(cluster=w271, "Action Name"="Perspective Change", "State Changed?"=TRUE) -> (w270:T4)
            n88 = Bundle By Name(cluster=w279, "Grabbing?"=FALSE) -> (w278:T7)
          }
        }
      }
      event "Main Graph": Mouse Leave {
        n89 = event-data() -> ()  [unwired: 1 in, 1 out]
        n90 = Unbundle By Name(w287) -> ("Grabbing?"=w286:bool)
        n91 = case shown="True" w286 {
          tunnel: [w293 w305] -> w288
          tunnel: w287 -> [w293 w304]
          tunnel: w285 -> [_ w299]
          tunnel: w284 -> [w292 w298]
          tunnel: [w292 w297] -> w283
          tunnel: [w291 w294] -> w282
          frame False {
            w291 = T8[] [] items=["[Data] Default", "[Data] Update Graph", "[Pane] Calculate Size from Coord Change", "[Pane] Calculate Size from Display State", "[Plot] Redraw Frame", "[Plot] Update Plot Color", "[Scale] Autoscale or Crop X, Y, Z", "[Scale] Resize Scales", "[Scale] Align Scale Labels", "[Plot] Initialize Plot", "[Scale] X Scale", "[Scale] Y Scale", "[Scale] Z Scale", "[Scale] Multiplier/Offset", "[Scale] Name", "[Scale] Visible", "[Scale] Label Visible", "[Scale] Format"] ("element")
          }
          frame True {
            w294 = T8[] [enum."[Pane] Calculate Size from Coord Change", enum."[Scale] Resize Scales", enum."[Scale] Align Scale Labels", enum."[Plot] Redraw Frame", enum."[Data] Update Graph"] items=["[Data] Default", "[Data] Update Graph", "[Pane] Calculate Size from Coord Change", "[Pane] Calculate Size from Display State", "[Plot] Redraw Frame", "[Plot] Update Plot Color", "[Scale] Autoscale or Crop X, Y, Z", "[Scale] Resize Scales", "[Scale] Align Scale Labels", "[Plot] Initialize Plot", "[Scale] X Scale", "[Scale] Y Scale", "[Scale] Z Scale", "[Scale] Multiplier/Offset", "[Scale] Name", "[Scale] Visible", "[Scale] Label Visible", "[Scale] Format"] ("element")
            n92 = Unbundle By Name(w299) -> ("Refnum"=w302:refnum<vi>)
            n93 = property class="Ctl"(reference=w302) -> ("OwningVI"=w301:refnum<vi>)  [unwired: 1 in, 2 out]
            n94 = Bundle By Name(cluster=w304, "Grabbing?"=FALSE) -> (w305:T7)
            n95 = call-poly <vilib>:"Set Cursor.vi"("VI reference (current VI)"=w301, "icon"=u16 0) -> ()  [unwired: 8 in, 2 out]
            n96 = Bundle By Name(cluster=w298, "Action Name"="Perspective Change", "State Changed?"=TRUE) -> (w297:T4)
          }
        }
      }
      event "background": Mouse Down? {
        n97 = event-data() -> ()  [unwired: 1 in, 1 out]
        n98 = event-data() -> ()  [unwired: 2 in, 1 out]
        "background" <- FALSE ("background")
      }
      event "background": Mouse Up {
        # "attempt to save color if they apply paint brush without opening color palette"
        n99 = event-data() -> ()  [unwired: 1 in, 8 out]
        n100 = property on="background" class="Bool"() -> ("Colors [4]"=w317:cluster{u32, u32}[])  [unwired: 2 in, 2 out]
        n101 = Index Array(array=w317) -> (element=w318:cluster{u32, u32})  [unwired: 1 in]
        n102 = Unbundle(w318) -> (w319:u32)  [unwired: 1 out]
        n103 = Unbundle By Name(w315) -> ("Decor color"=w316:u32)
        n104 = Not Equal?(x=w316, y=w319) -> (x != y?=w311:bool)
        n105 = Bundle By Name(cluster=w315, "Decor color"=w319) -> (w314:T5)
        n106 = Bundle By Name(cluster=w313, "State Changed?"=w311) -> (w312:T4)
      }
      event "XY Scale Graph": Scale Range Change {
        w328 = T8[] [enum."[Scale] Autoscale or Crop X, Y, Z", enum."[Data] Update Graph"] items=["[Data] Default", "[Data] Update Graph", "[Pane] Calculate Size from Coord Change", "[Pane] Calculate Size from Display State", "[Plot] Redraw Frame", "[Plot] Update Plot Color", "[Scale] Autoscale or Crop X, Y, Z", "[Scale] Resize Scales", "[Scale] Align Scale Labels", "[Plot] Initialize Plot", "[Scale] X Scale", "[Scale] Y Scale", "[Scale] Z Scale", "[Scale] Multiplier/Offset", "[Scale] Name", "[Scale] Visible", "[Scale] Label Visible", "[Scale] Format"] ("element")
        n107 = Unbundle By Name(w325) -> ("Scale Range Change"=w322:refnum<user-event>, "out of state queue"=w327:refnum<queue>)
        n108 = event-data() -> ("NewRange.Maximum"=w335:dbl, "NewRange.Minimum"=w334:dbl, "Kind"=w340:enum16{"X-Scale", "Y-Scale", "Z-Scale"})  [unwired: 1 in]
        n109 = Dequeue Element(queue=w327) -> (queue out=w323:refnum<queue>, element=w326:T9)  [unwired: 2 in, 2 out]
        n110 = case shown="\"X-Scale\", Default" w340 {
          tunnel: w325 -> [w355 w368]
          tunnel: [w351 w369] -> w324
          tunnel: w335 -> [w342 w359]
          tunnel: w334 -> [w343 w358]
          tunnel: [w350 w363] -> w332
          tunnel: [w349 w364] -> w331
          tunnel: [enum16{"X-Scale", "Y-Scale", "Z-Scale"}."X-Scale" ("Kind") enum16{"X-Scale", "Y-Scale", "Z-Scale"}."Y-Scale" ("Kind")] -> w330
          tunnel: w326 -> [w352 w365]
          frame "X-Scale", Default {
            n111 = Unbundle By Name(w355) -> ("X-Axis Scaling Factor.Multiplier"=w345:dbl, "X-Axis Scaling Factor.Offset"=w344:dbl)
            n112 = call <vilib>:"svx_Oct_Waterfall XYZ Scale.vi"("Minimum"=w343, "Maximum"=w342, "Offset"=w344, "Multiplier"=w345) -> ("Scaled.Minimum"=w350:dbl, "Scaled.Maximum"=w349:dbl, "Range.Minimum"=w347:dbl, "Range.Maximum"=w348:dbl, "flipped?"=w346:bool)  [unwired: 3 in]
            n113 = property on="XY Scale Graph" class="WFGraph (strict)"("XScale.Flipped"=w346) -> ()  [unwired: 2 in, 2 out]
            n114 = Bundle By Name(cluster=w352, "AutoScale X"=u8 0, "X-Axis Range.Maximum"=w348, "X-Axis Range.Minimum"=w347, "X-Axis Range Scaled.Minimum"=w350, "X-Axis Range Scaled.Maximum"=w349) -> (w351:T9)
          }
          frame "Y-Scale" {
            n115 = Unbundle By Name(w368) -> ("Y-Axis Scaling Factor.Multiplier"=w357:dbl, "Y-Axis Scaling Factor.Offset"=w356:dbl)
            n116 = call <vilib>:"svx_Oct_Waterfall XYZ Scale.vi"("Minimum"=w358, "Maximum"=w359, "Offset"=w356, "Multiplier"=w357) -> ("Scaled.Minimum"=w363:dbl, "Scaled.Maximum"=w364:dbl, "Range.Minimum"=w361:dbl, "Range.Maximum"=w362:dbl, "flipped?"=w360:bool)  [unwired: 3 in]
            n117 = property on="XY Scale Graph" class="WFGraph (strict)"("YScale.Flipped"=w360) -> ()  [unwired: 2 in, 2 out]
            n118 = Bundle By Name(cluster=w365, "AutoScale Y"=u8 0, "Y-Axis Range.Maximum"=w362, "Y-Axis Range.Minimum"=w361, "Y-Axis Range Scaled.Minimum"=w363, "Y-Axis Range Scaled.Maximum"=w364) -> (w369:T9)
          }
        }
        n119 = Bundle By Name(cluster=w339, "Action Name"="Range Change", "State Changed?"=TRUE) -> (w338:T4)
        n120 = Bundle("Scaled.Minimum"=w332, "Scaled.Maximum"=w331, "Kind"=w330) -> (w333:T10)  [unwired: 1 in]
        n121 = Enqueue Element(queue=w323, element=w324) -> ()  [unwired: 2 in, 3 out]
        n122 = Generate User Event(user event=w322, event data cluster=w333) -> ()  [unwired: 2 in, 2 out]
      }
      event "Z Scale Graph": Scale Range Change {
        w370 = T8[] [enum."[Scale] Autoscale or Crop X, Y, Z", enum."[Data] Update Graph"] items=["[Data] Default", "[Data] Update Graph", "[Pane] Calculate Size from Coord Change", "[Pane] Calculate Size from Display State", "[Plot] Redraw Frame", "[Plot] Update Plot Color", "[Scale] Autoscale or Crop X, Y, Z", "[Scale] Resize Scales", "[Scale] Align Scale Labels", "[Plot] Initialize Plot", "[Scale] X Scale", "[Scale] Y Scale", "[Scale] Z Scale", "[Scale] Multiplier/Offset", "[Scale] Name", "[Scale] Visible", "[Scale] Label Visible", "[Scale] Format"] ("element")
        # "True = Z Scale should\nbe flipped"
        # "If user flips scale from how the scale should be,\nflip the data."
        n123 = event-data() -> ("NewRange.Maximum"=w375:dbl, "NewRange.Minimum"=w374:dbl)  [unwired: 1 in]
        n124 = Unbundle By Name(w399) -> ("dz"=w394:dbl)
        n125 = Unbundle By Name(w385) -> ("out of state queue"=w382:refnum<queue>, "Z-Axis Scaling Factor.Multiplier"=w377:dbl, "Z-Axis Scaling Factor.Offset"=w376:dbl, "Rev Z Order"=w393:bool, "Scale Range Change"=w383:refnum<user-event>)
        n126 = Dequeue Element(queue=w382) -> (queue out=w372:refnum<queue>, element=w373:T9)  [unwired: 2 in, 2 out]
        n127 = call <vilib>:"svx_Oct_Waterfall XYZ Scale.vi"("Minimum"=w374, "Maximum"=w375, "Offset"=w376, "Multiplier"=w377) -> ("Scaled.Minimum"=w378:dbl, "Scaled.Maximum"=w379:dbl, "Range.Minimum"=w380:dbl, "Range.Maximum"=w381:dbl)  [unwired: 3 in, 1 out]
        n128 = Less Than 0?(x=w394) -> (x < 0?=w391:bool)
        n129 = Bundle By Name(cluster=w373, "AutoScale Z"=u8 0, "Z-Axis Range.Maximum"=w381, "Z-Axis Range.Minimum"=w380, "Z-Axis Range Scaled.Maximum"=w379, "Z-Axis Range Scaled.Minimum"=w378) -> (w371:T9)
        n130 = Subtract(x=w375, y=w374) -> (x-y=w398:dbl)
        n131 = Exclusive Or(1:w393, 2:w391) -> (0:w392:bool)
        n132 = Less Than 0?(x=w398) -> (x < 0?=w397:bool)
        n133 = Bundle("Range.Minimum"=w380, "Range.Maximum"=w381, "Kind"=enum16{"X-Scale", "Y-Scale", "Z-Scale"}."Z-Scale") -> (w387:T11)  [unwired: 1 in]
        n134 = Equal?(x=w392, y=w397) -> (x = y?=w396:bool)
        n135 = Generate User Event(user event=w383, event data cluster=w387) -> ()  [unwired: 2 in, 2 out]
        n136 = Not(x=w393) -> (.not. x?=w395:bool)
        n137 = Select(t=w393, s=w396, f=w395) -> (s? t:f=w384:bool)
        n138 = Enqueue Element(queue=w372, element=w371) -> ()  [unwired: 2 in, 3 out]
        n139 = Bundle By Name(cluster=w401, "Action Name"="Range Change", "State Changed?"=TRUE) -> (w400:T4)
        n140 = Bundle By Name(cluster=w385, "Rev Z Order"=w384) -> (w386:T5)
      }
      event Pane Size {
        w404 = T8[] [enum."[Pane] Calculate Size from Display State", enum."[Scale] Resize Scales", enum."[Scale] Align Scale Labels", enum."[Plot] Redraw Frame", enum."[Data] Update Graph"] items=["[Data] Default", "[Data] Update Graph", "[Pane] Calculate Size from Coord Change", "[Pane] Calculate Size from Display State", "[Plot] Redraw Frame", "[Plot] Update Plot Color", "[Scale] Autoscale or Crop X, Y, Z", "[Scale] Resize Scales", "[Scale] Align Scale Labels", "[Plot] Initialize Plot", "[Scale] X Scale", "[Scale] Y Scale", "[Scale] Z Scale", "[Scale] Multiplier/Offset", "[Scale] Name", "[Scale] Visible", "[Scale] Label Visible", "[Scale] Format"] ("element")
        n141 = event-data() -> ("NewBnds"=w408:T12)  [unwired: 1 in]
        n142 = stacked-sequence {
          tunnel: w408 -> [_ w419 _]
          frame #0 {
            n143 = control-ref of="This VI"() -> (w410:refnum<vi>)
            n144 = property class="FcdVI"(reference=w410) -> (error out=w411:errorcluster, "Panel"=w413:refnum<vi>)  [unwired: 1 in, 1 out]
            n145 = property class="Pnl"(reference=w413, error in=w411, "DeferPanUpdts"=TRUE ("Defer Panel Updates")) -> ()  [unwired: 2 out]
          }
          frame #1 {
            # "-1 because 3D box was being cutoff by one pixel at the bottom"
            n146 = Unbundle By Name(w419) -> ("Right"=w420:i16, "Left"=w421:i16, "Bottom"=w422:i16, "Top"=w423:i16)
            n147 = Subtract(x=w420, y=w421) -> (x-y=w415:i16)
            n148 = Subtract(x=w422, y=w423) -> (x-y=w416:i16)
            n149 = Subtract(x=w415, y=i16 150 ("Width Offset")) -> (x-y=w418:i16)
            n150 = Subtract(x=w416, y=i16 60 ("Height Offset")) -> (x-y=w417:i16)
            n151 = Decrement(x=w416) -> (x-1=w414:i16)
            n152 = property on="Main Graph" class="XYGraph (strict)"("Width"=w418, "Height"=w417) -> ()  [unwired: 2 in, 2 out]
            n153 = property on="background" class="Bool"("Width"=w415, "Height"=w414) -> ()  [unwired: 2 in, 2 out]
          }
          frame #2 {
            # "Reposition Scales"
            n154 = property on="XY Scale Graph" class="WFGraph (strict)"() -> ("Plot Bounds"=w444:T12, "Position"=w438:T13)  [unwired: 2 in, 2 out]
            n155 = property on="Main Graph" class="XYGraph (strict)"() -> ("Plot Bounds"=w445:T12)  [unwired: 2 in, 2 out]
            n156 = property on="Z Scale Graph" class="WFGraph (strict)"() -> ("Position"=w428:T13, "Plot Bounds"=w433:T12)  [unwired: 2 in, 2 out]
            n157 = Unbundle By Name(w445) -> ("Right"=w435:i16, "Left"=w436:i16, "Bottom"=w434:i16)
            n158 = Unbundle By Name(w444) -> ("Left"=w443:i16, "Bottom"=w442:i16)
            n159 = Unbundle By Name(w433) -> ("Right"=w432:i16, "Bottom"=w431:i16)
            n160 = Bundle("Right"=w432, "Bottom"=w431) -> (w430:cluster{"Right":i16, "Bottom":i16})  [unwired: 1 in]
            n161 = Bundle("Right"=w435, "Bottom"=w434) -> (w429:cluster{"Right":i16, "Bottom":i16})  [unwired: 1 in]
            n162 = Bundle("Left"=w436, "Bottom"=w434) -> (w441:cluster{"Left":i16, "Bottom":i16})  [unwired: 1 in]
            n163 = Bundle("Left"=w443, "Bottom"=w442) -> (w440:cluster{"Left":i16, "Bottom":i16})  [unwired: 1 in]
            n164 = Subtract(x=w430, y=w429) -> (x-y=w427:cluster{"Right":i16, "Bottom":i16})
            n165 = Subtract(x=w441, y=w440) -> (x-y=w439:cluster{"Left":i16, "Bottom":i16})
            n166 = Subtract(x=w428, y=w427) -> (x-y=w426:T13)
            n167 = Add(x=w439, y=w438) -> (x+y=w437:T13)
            n168 = property on="Z Scale Graph" class="WFGraph (strict)"("Position"=w426) -> ()  [unwired: 2 in, 2 out]
            n169 = property on="XY Scale Graph" class="WFGraph (strict)"("Position"=w437) -> ()  [unwired: 2 in, 2 out]
          }
        }
      }
      event "Z Scale Graph", "Main Graph", "XY Scale Graph": Shortcut Menu Activation? {
        n170 = event-data() -> ("Coords"=→"Coords":T1, "CtlRef"=w452:refnum<vi>, "MenuRef"=w450:refnum<k9>)  [unwired: 1 in]
        n171 = control-ref of="Main Graph"() -> (w451:refnum<vi>)
        n172 = Not Equal?(x=w451, y=w452) -> (x != y?=w449:bool)
        n173 = call <vilib>:"svx_Oct_Waterfall Shortcut Menu.vi"("main graph?"=w449, "Container State"=w448, "State"=w447, "menu reference in"=w450) -> ()  [unwired: 7 in, 1 out]
        n174 = event-data() -> ()  [unwired: 2 in, 1 out]
      }
      event Shortcut Menu Activation? {
        # "Delete unwanted menu items"
        n175 = event-data() -> ("MenuRef"=w457:refnum<k9>)  [unwired: 1 in]
        n176 = for {
          tunnel: cluster{"menu tag":string, string[]}[] [{"menu tag"="APP_SC_ADVANCED", ["APP_SC_KEY_NAVIGATION", "APP_SC_CUSTOMIZE", "APP_SC_SHOW_DIAGRAM"]}, {"menu tag"="", ["APP_SC_PROPERTIES", "APP_SC_SHOW_DIAGRAM"]}] -> [w468] mode=indexing
          shift-right: [w465] -> w456
          shift-left: w457 -> [w469]
          n177 = Unbundle(w468) -> ("menu tag"=w467:string, w466:string[])
          n178 = Delete Menu Items(7:w466, 8:w467, 9:w469) -> (3:w465:refnum<k9>)  [unwired: 1 in, 1 out]
        }
        n179 = Unbundle By Name(w460) -> ("Run Mode?"=w459:bool)
        n180 = case shown="False" w459 {
          tunnel: w456 -> [w470 _]
          frame False {
            n181 = Insert Menu Items(7:string[] ["SV_WF_PROPERTIES"], 8:string[] ["Properties"], 9:w470) -> ()  [unwired: 3 in, 3 out]
          }
          frame True {
          }
        }
        n182 = event-data() -> ()  [unwired: 2 in, 1 out]
      }
      event "Z Scale Graph", "Main Graph", "XY Scale Graph": Shortcut Menu Selection (User) {
        n183 = event-data() -> ("ItemTag"=w481:string)  [unwired: 1 in]
        n184 = case shown="Default" w481 {
          tunnel: w479 -> [w482 w490 w500 w510 w516 w534 w552 w572 w585 w593 w608 w617]
          tunnel: [w482 w489 w499 w509 w516 w534 w552 w570 w586 w594 w608 w617] -> w478
          tunnel: [w483 w491 w501 w511 w530 w547 w566 w577 w588 w607 w616 w625] -> w476
          tunnel: w477 -> [w483 w492 w502 w512 w531 w548 w565 w576 w587 w606 w615 w624]
          tunnel: w475 -> [_ _ _ _ _ _ _ _ _ w605 _ _]
          tunnel: w474 -> [_ _ _ _ _ _ _ _ _ w604 w614 w623]
          tunnel: [_ _ _ _ w515 w537 w555 w568 w579 w596 _ _] -> w473
          frame Default {
          }
          frame "SV_WF_VISIBLE_ITEMS_X_SCALE" {
            n185 = Unbundle By Name(w490) -> ("X-Scale Visible"=w488:bool)
            n186 = Not(x=w488) -> (.not. x?=w484:bool)
            n187 = Bundle By Name(cluster=w490, "X-Scale Visible"=w484) -> (w489:T5)
            n188 = property on="XY Scale Graph" class="WFGraph (strict)"("XScale.Visible"=w484) -> ()  [unwired: 2 in, 2 out]
            n189 = Select(t="Show X Scale" ("Action Name"), s=w484, f="Hide X Scale") -> (s? t:f=w485:string)
            n190 = Bundle By Name(cluster=w492, "Action Name"=w485, "State Changed?"=TRUE) -> (w491:T4)
          }
          frame "SV_WF_VISIBLE_ITEMS_Y_SCALE" {
            n191 = Unbundle By Name(w500) -> ("Y-Scale Visible"=w498:bool)
            n192 = Not(x=w498) -> (.not. x?=w494:bool)
            n193 = Bundle By Name(cluster=w500, "Y-Scale Visible"=w494) -> (w499:T5)
            n194 = property on="XY Scale Graph" class="WFGraph (strict)"("YScale.Visible"=w494) -> ()  [unwired: 2 in, 2 out]
            n195 = Select(t="Show Y Scale" ("Action Name"), s=w494, f="Hide Y Scale") -> (s? t:f=w495:string)
            n196 = Bundle By Name(cluster=w502, "Action Name"=w495, "State Changed?"=TRUE) -> (w501:T4)
          }
          frame "SV_WF_VISIBLE_ITEMS_Z_SCALE" {
            n197 = Unbundle By Name(w510) -> ("Z-Scale Visible"=w508:bool)
            n198 = Not(x=w508) -> (.not. x?=w505:bool)
            n199 = Bundle By Name(cluster=w510, "Z-Scale Visible"=w505) -> (w509:T5)
            n200 = property on="Z Scale Graph" class="WFGraph (strict)"("YScale.Visible"=w505) -> ()  [unwired: 2 in, 2 out]
            n201 = Select(t="Show Z Scale" ("Action Name"), s=w505, f="Hide Z Scale") -> (s? t:f=w506:string)
            n202 = Bundle By Name(cluster=w512, "Action Name"=w506, "State Changed?"=TRUE) -> (w511:T4)
          }
          frame "SV_WF_AUTOSCALE_X" {
            w515 = T8[] [enum."[Scale] Autoscale or Crop X, Y, Z", enum."[Data] Update Graph"] items=["[Data] Default", "[Data] Update Graph", "[Pane] Calculate Size from Coord Change", "[Pane] Calculate Size from Display State", "[Plot] Redraw Frame", "[Plot] Update Plot Color", "[Scale] Autoscale or Crop X, Y, Z", "[Scale] Resize Scales", "[Scale] Align Scale Labels", "[Plot] Initialize Plot", "[Scale] X Scale", "[Scale] Y Scale", "[Scale] Z Scale", "[Scale] Multiplier/Offset", "[Scale] Name", "[Scale] Visible", "[Scale] Label Visible", "[Scale] Format"] ("element")
            n203 = Unbundle By Name(w516) -> ("out of state queue"=w519:refnum<queue>)
            n204 = Dequeue Element(queue=w519) -> (queue out=w518:refnum<queue>, element=w514:T9)  [unwired: 2 in, 2 out]
            n205 = Unbundle By Name(w514) -> ("AutoScale X"=w525:u8)
            n206 = Equal?(x=w525, y=u8 2) -> (x = y?=w520:bool)
            n207 = Select(t=u8 0 ("y"), s=w520, f=u8 2 ("y")) -> (s? t:f=w524:u8)
            n208 = Select(t="Autoscale Deselection" ("Action Name"), s=w520, f="Autoscale Selection") -> (s? t:f=w521:string)
            n209 = Bundle By Name(cluster=w531, "Action Name"=w521, "State Changed?"=TRUE) -> (w530:T4)
            n210 = Bundle By Name(cluster=w514, "AutoScale X"=w524) -> (w517:T9)
            n211 = Enqueue Element(queue=w518, element=w517) -> ()  [unwired: 2 in, 3 out]
          }
          frame "SV_WF_AUTOSCALE_Y" {
            w537 = T8[] [enum."[Scale] Autoscale or Crop X, Y, Z", enum."[Data] Update Graph"] items=["[Data] Default", "[Data] Update Graph", "[Pane] Calculate Size from Coord Change", "[Pane] Calculate Size from Display State", "[Plot] Redraw Frame", "[Plot] Update Plot Color", "[Scale] Autoscale or Crop X, Y, Z", "[Scale] Resize Scales", "[Scale] Align Scale Labels", "[Plot] Initialize Plot", "[Scale] X Scale", "[Scale] Y Scale", "[Scale] Z Scale", "[Scale] Multiplier/Offset", "[Scale] Name", "[Scale] Visible", "[Scale] Label Visible", "[Scale] Format"] ("element")
            n212 = Unbundle By Name(w534) -> ("out of state queue"=w536:refnum<queue>)
            n213 = Dequeue Element(queue=w536) -> (queue out=w535:refnum<queue>, element=w532:T9)  [unwired: 2 in, 2 out]
            n214 = Unbundle By Name(w532) -> ("AutoScale Y"=w546:u8)
            n215 = Equal?(x=w546, y=u8 2) -> (x = y?=w539:bool)
            n216 = Select(t=u8 0 ("y"), s=w539, f=u8 2 ("y")) -> (s? t:f=w542:u8)
            n217 = Select(t="Autoscale Deselection" ("Action Name"), s=w539, f="Autoscale Selection") -> (s? t:f=w538:string)
            n218 = Bundle By Name(cluster=w532, "AutoScale Y"=w542) -> (w533:T9)
            n219 = Bundle By Name(cluster=w548, "Action Name"=w538, "State Changed?"=TRUE) -> (w547:T4)
            n220 = Enqueue Element(queue=w535, element=w533) -> ()  [unwired: 2 in, 3 out]
          }
          frame "SV_WF_AUTOSCALE_Z" {
            w555 = T8[] [enum."[Scale] Autoscale or Crop X, Y, Z", enum."[Data] Update Graph"] items=["[Data] Default", "[Data] Update Graph", "[Pane] Calculate Size from Coord Change", "[Pane] Calculate Size from Display State", "[Plot] Redraw Frame", "[Plot] Update Plot Color", "[Scale] Autoscale or Crop X, Y, Z", "[Scale] Resize Scales", "[Scale] Align Scale Labels", "[Plot] Initialize Plot", "[Scale] X Scale", "[Scale] Y Scale", "[Scale] Z Scale", "[Scale] Multiplier/Offset", "[Scale] Name", "[Scale] Visible", "[Scale] Label Visible", "[Scale] Format"] ("element")
            n221 = Unbundle By Name(w552) -> ("out of state queue"=w554:refnum<queue>)
            n222 = Dequeue Element(queue=w554) -> (queue out=w553:refnum<queue>, element=w550:T9)  [unwired: 2 in, 2 out]
            n223 = Unbundle By Name(w550) -> ("AutoScale Z"=w561:u8)
            n224 = Equal?(x=w561, y=u8 2) -> (x = y?=w556:bool)
            n225 = Select(t=u8 0 ("y"), s=w556, f=u8 2 ("y")) -> (s? t:f=w560:u8)
            n226 = Select(t="Autoscale Deselection" ("Action Name"), s=w556, f="Autoscale Selection") -> (s? t:f=w557:string)
            n227 = Bundle By Name(cluster=w550, "AutoScale Z"=w560) -> (w551:T9)
            n228 = Bundle By Name(cluster=w565, "Action Name"=w557, "State Changed?"=TRUE) -> (w566:T4)
            n229 = Enqueue Element(queue=w553, element=w551) -> ()  [unwired: 2 in, 3 out]
          }
          frame "SV_WF_PLOT_TRANSPARENCY" {
            w568 = T8[] [enum."[Plot] Update Plot Color"] items=["[Data] Default", "[Data] Update Graph", "[Pane] Calculate Size from Coord Change", "[Pane] Calculate Size from Display State", "[Plot] Redraw Frame", "[Plot] Update Plot Color", "[Scale] Autoscale or Crop X, Y, Z", "[Scale] Resize Scales", "[Scale] Align Scale Labels", "[Plot] Initialize Plot", "[Scale] X Scale", "[Scale] Y Scale", "[Scale] Z Scale", "[Scale] Multiplier/Offset", "[Scale] Name", "[Scale] Visible", "[Scale] Label Visible", "[Scale] Format"] ("element")
            n230 = Unbundle By Name(w572) -> ("Plot Transparency"=w569:bool)
            n231 = Select(t="Plot Transparency Deselection" ("Action Name"), s=w569, f="Plot Transparency Selection") -> (s? t:f=w573:string)
            n232 = Not(x=w569) -> (.not. x?=w571:bool)
            n233 = Bundle By Name(cluster=w576, "Action Name"=w573, "State Changed?"=TRUE) -> (w577:T4)
            n234 = Bundle By Name(cluster=w572, "Plot Transparency"=w571) -> (w570:T5)
          }
          frame "SV_REVERSE_ORDER" {
            w579 = T8[] [enum."[Scale] Autoscale or Crop X, Y, Z", enum."[Data] Update Graph"] items=["[Data] Default", "[Data] Update Graph", "[Pane] Calculate Size from Coord Change", "[Pane] Calculate Size from Display State", "[Plot] Redraw Frame", "[Plot] Update Plot Color", "[Scale] Autoscale or Crop X, Y, Z", "[Scale] Resize Scales", "[Scale] Align Scale Labels", "[Plot] Initialize Plot", "[Scale] X Scale", "[Scale] Y Scale", "[Scale] Z Scale", "[Scale] Multiplier/Offset", "[Scale] Name", "[Scale] Visible", "[Scale] Label Visible", "[Scale] Format"] ("element")
            n235 = Unbundle By Name(w585) -> ("Rev Z Order"=w580:bool)
            n236 = Not(x=w580) -> (.not. x?=w584:bool)
            n237 = Select(t="Reverse Order Deselection" ("Action Name"), s=w580, f="Reverse Order Selection") -> (s? t:f=w581:string)
            n238 = Bundle By Name(cluster=w585, "Rev Z Order"=w584) -> (w586:T5)
            n239 = Bundle By Name(cluster=w587, "Action Name"=w581, "State Changed?"=TRUE) -> (w588:T4)
          }
          frame "SV_WF_PROPERTIES" {
            w596 = T8[] [enum."[Scale] Autoscale or Crop X, Y, Z", enum."[Data] Update Graph"] items=["[Data] Default", "[Data] Update Graph", "[Pane] Calculate Size from Coord Change", "[Pane] Calculate Size from Display State", "[Plot] Redraw Frame", "[Plot] Update Plot Color", "[Scale] Autoscale or Crop X, Y, Z", "[Scale] Resize Scales", "[Scale] Align Scale Labels", "[Plot] Initialize Plot", "[Scale] X Scale", "[Scale] Y Scale", "[Scale] Z Scale", "[Scale] Multiplier/Offset", "[Scale] Name", "[Scale] Visible", "[Scale] Label Visible", "[Scale] Format"] ("element")
            n240 = call <vilib>:"svx_Oct_Waterfall QueueToState.vi"("State In"=w593) -> ("State Out"=w592:T5)  [unwired: 10 in]
            n241 = Unbundle By Name(w604) -> ("Refnum"=w603:refnum<vi>)
            n242 = control-ref of="XY Scale Graph"() -> (w602:refnum<vi>)
            n243 = control-ref of="Z Scale Graph"() -> (w601:refnum<vi>)
            n244 = local read "# Plots Updated"() -> (w591:i32)
            n245 = control-ref of="Main Graph"() -> (w600:refnum<vi>)
            n246 = call <vilib>:"svx_Oct_Property Page.vi"("# Plots Updated in"=w591, "Z Scale Graph Refnum"=w601, "Main Graph"=w600, "XY Scale Graph Refnum"=w602, "Container Refnum"=w603, "State in"=w592, "Data In"=w605) -> ("# Plots Updated out"=w590:i32, "Cancel?"=w598:bool, "State out"=w595:T5)  [unwired: 2 in]
            n247 = local write "# Plots Updated"(w590) -> ()
            n248 = Not(x=w598) -> (.not. x?=w599:bool)
            n249 = Bundle By Name(cluster=w606, "Action Name"="Property Page Changes", "State Changed?"=w599) -> (w607:T4)
            n250 = call <vilib>:"svx_Oct_Waterfall StateToQueue.vi"("State In"=w595) -> ("State Out"=w594:T5)  [unwired: 10 in]
          }
          frame "APP_SC_LABEL" {
            n251 = Unbundle By Name(w614) -> ("Refnum"=w609:refnum<vi>)
            n252 = property class="Ctl"(reference=w609) -> (reference out=w612:refnum<vi>, "Label.Visible"=w610:bool)  [unwired: 1 in, 1 out]
            n253 = Not(x=w610) -> (.not. x?=w611:bool)
            n254 = property class="Ctl"(reference=w612, "Label.Visible"=w611) -> ()  [unwired: 1 in, 2 out]
            n255 = Bundle By Name(cluster=w615, "Action Name"="Label Visability") -> (w616:T4)
          }
          frame "APP_SC_CAPTION" {
            n256 = Unbundle By Name(w623) -> ("Refnum"=w618:refnum<vi>)
            n257 = property class="Ctl"(reference=w618) -> (reference out=w621:refnum<vi>, "Caption.Visible"=w619:bool)  [unwired: 1 in, 1 out]
            n258 = Not(x=w619) -> (.not. x?=w620:bool)
            n259 = property class="Ctl"(reference=w621, "Caption.Visible"=w620) -> ()  [unwired: 1 in, 2 out]
            n260 = Bundle By Name(cluster=w624, "Action Name"="Caption Visability") -> (w625:T4)
          }
        }
      }
      event "XY Scale Graph", "Z Scale Graph", "Main Graph": Shortcut Menu Selection? (App) {
        n261 = event-data() -> ("ItemTag"=w633:string, "Coords"=w626:T1)  [unwired: 1 in]
        n262 = local write "Coords"(w626) -> ()
        n263 = case shown="\"APP_SC_CLEAR_GRAPH\"" w633 {
          tunnel: [FALSE ("Discard?") TRUE ("Discard?")] -> w634
          tunnel: w632 -> [w638 _]
          tunnel: [w638 T2 {"z0"=0.0, "dz"=1.0, "Plots"=[]} ("Data In")] -> w631
          tunnel: [w637 w645] -> w629
          tunnel: w630 -> [w637 w643]
          tunnel: [w636 w640] -> w627
          frame Default {
            w636 = T8[] [] items=["[Data] Default", "[Data] Update Graph", "[Pane] Calculate Size from Coord Change", "[Pane] Calculate Size from Display State", "[Plot] Redraw Frame", "[Plot] Update Plot Color", "[Scale] Autoscale or Crop X, Y, Z", "[Scale] Resize Scales", "[Scale] Align Scale Labels", "[Plot] Initialize Plot", "[Scale] X Scale", "[Scale] Y Scale", "[Scale] Z Scale", "[Scale] Multiplier/Offset", "[Scale] Name", "[Scale] Visible", "[Scale] Label Visible", "[Scale] Format"] ("element")
          }
          frame "APP_SC_CLEAR_GRAPH" {
            w640 = T8[] [enum."[Scale] Autoscale or Crop X, Y, Z", enum."[Data] Update Graph"] items=["[Data] Default", "[Data] Update Graph", "[Pane] Calculate Size from Coord Change", "[Pane] Calculate Size from Display State", "[Plot] Redraw Frame", "[Plot] Update Plot Color", "[Scale] Autoscale or Crop X, Y, Z", "[Scale] Resize Scales", "[Scale] Align Scale Labels", "[Plot] Initialize Plot", "[Scale] X Scale", "[Scale] Y Scale", "[Scale] Z Scale", "[Scale] Multiplier/Offset", "[Scale] Name", "[Scale] Visible", "[Scale] Label Visible", "[Scale] Format"] ("element")
            n264 = Bundle By Name(cluster=w643, "Action Name"="Clear Graph", "Data Changed?"=TRUE) -> (w645:T4)
          }
        }
        n265 = event-data("Discard?"=w634) -> ()  [unwired: 1 in, 1 out]
      }
      event Mouse Down? {
        n266 = event-data() -> ("Button"=w652:u16, "Mods"=w653:cluster{"Double Click":bool, "Menu Key":bool}, "PlatMods"=w650:T14, "Coords"=w647:T1)  [unwired: 1 in]
        n267 = case shown="1" w652 {
          tunnel: w653 -> [w663 w665]
          tunnel: [w664 w665] -> w651
          tunnel: w647 -> [w662 _]
          frame 1 {
            n268 = local read "Coords"() -> (w661:T1)
            n269 = Unbundle By Name(w663) -> ("Double Click"=w659:bool)
            n270 = Equal?(x=w662, y=w661) -> (x = y?=w660:bool)
            n271 = Select(t=FALSE ("Double Click"), s=w660, f=w659) -> (s? t:f=w657:bool)
            n272 = Bundle By Name(cluster=w663, "Double Click"=w657) -> (w664:cluster{"Double Click":bool, "Menu Key":bool})
          }
          frame 0, Default {
          }
        }
        n273 = event-data("Button"=w652, "Mods"=w651, "PlatMods"=w650, "Discard?"=FALSE) -> ()  [unwired: 1 in, 1 out]
      }
    }
    n274 = local read "# Plots Updated"() -> (w15:i32)
    n275 = local read "Dec/Cropped"() -> (w14:T2)
    n276 = control-ref of="XY Scale Graph"() -> (w10:refnum<vi>)
    n277 = control-ref of="Z Scale Graph"() -> (w9:refnum<vi>)
    n278 = control-ref of="Main Graph"() -> (w11:refnum<vi>)
    n279 = control-ref of="background"() -> (w8:refnum<vi>)
    n280 = control-ref of="This VI"() -> (w19:refnum<vi>)
    n281 = call <vilib>:"svx_Oct_Waterfall Execute.vi"("Data In"=w21, "Display State In"=w22, "Container State"=w17, "# Plots Updated"=w15, "Dec/Cropped in"=w14, "Execution Tasks"=w23, "Main Graph"=w11, "Coords"=w18, "XY Scale Graph ref"=w10, "Z Scale Graph ref"=w9, "This VI"=w19, "Background ref"=w8) -> ("Data Out"=w20:T2, "Display State Out"=w12:T5, "# Plots Updated out"=→"# Plots Updated":i32, "Dec/Cropped out"=→"Dec/Cropped":T2)  [unwired: 4 in]
  }
  "Display State Out" <- w4
  "Data Out" <- w7
  "Action" <- w2
  n282 = disable-structure shown="Disabled" {
    frame Disabled {
      # "Temporarily enable and run VI to reposition graphs"
      n283 = stacked-sequence {
        frame #0 {
          # "-1 because 3D box was being cutoff by one pixel at the bottom"
          n284 = property on="Pane" class="Pane"() -> ("Width"=w667:u32, "Height"=w666:u32)  [unwired: 2 in, 2 out]
          n285 = control-ref of="This VI"() -> (w671:refnum<vi>)
          n286 = property on="Property Node" class="FcdVI"(reference=w671) -> ("Panel"=w672:refnum<vi>)  [unwired: 1 in, 2 out]
          n287 = property on="Property Node" class="Pnl"(reference=w672) -> ("Decos[]"=w670:refnum<vi>[])  [unwired: 1 in, 2 out]
          n288 = Subtract(x=w667, y=i16 150 ("Width Offset")) -> (x-y=w674:u32)
          n289 = Subtract(x=w666, y=i16 60 ("Height Offset")) -> (x-y=w673:u32)
          n290 = Decrement(x=w666) -> (x-1=w668:u32)
          n291 = Index Array(array=w670) -> (element=w669:refnum<vi>)  [unwired: 1 in]
          n292 = property on="Main Graph" class="XYGraph (strict)"("Width"=w674, "Height"=w673) -> ()  [unwired: 2 in, 2 out]
          n293 = property on="Property Node" class="Decor"(reference=w669, "Width"=w667, "Height"=w668) -> ()  [unwired: 1 in, 2 out]
        }
        frame #1 {
          # "Reposition Scales"
          n294 = property on="XY Scale Graph" class="WFGraph (strict)"() -> ("Plot Bounds"=w695:T12, "Position"=w689:T13)  [unwired: 2 in, 2 out]
          n295 = property on="Main Graph" class="XYGraph (strict)"() -> ("Plot Bounds"=w696:T12)  [unwired: 2 in, 2 out]
          n296 = property on="Z Scale Graph" class="WFGraph (strict)"() -> ("Position"=w679:T13, "Plot Bounds"=w684:T12)  [unwired: 2 in, 2 out]
          n297 = Unbundle By Name(w696) -> ("Right"=w686:i16, "Left"=w687:i16, "Bottom"=w685:i16)
          n298 = Unbundle By Name(w695) -> ("Left"=w694:i16, "Bottom"=w693:i16)
          n299 = Unbundle By Name(w684) -> ("Right"=w683:i16, "Bottom"=w682:i16)
          n300 = Bundle("Right"=w683, "Bottom"=w682) -> (w681:cluster{"Right":i16, "Bottom":i16})  [unwired: 1 in]
          n301 = Bundle("Right"=w686, "Bottom"=w685) -> (w680:cluster{"Right":i16, "Bottom":i16})  [unwired: 1 in]
          n302 = Bundle("Left"=w687, "Bottom"=w685) -> (w692:cluster{"Left":i16, "Bottom":i16})  [unwired: 1 in]
          n303 = Bundle("Left"=w694, "Bottom"=w693) -> (w691:cluster{"Left":i16, "Bottom":i16})  [unwired: 1 in]
          n304 = Subtract(x=w681, y=w680) -> (x-y=w678:cluster{"Right":i16, "Bottom":i16})
          n305 = Subtract(x=w692, y=w691) -> (x-y=w690:cluster{"Left":i16, "Bottom":i16})
          n306 = Subtract(x=w679, y=w678) -> (x-y=w677:T13)
          n307 = Add(x=w690, y=w689) -> (x+y=w688:T13)
          n308 = property on="Z Scale Graph" class="WFGraph (strict)"("Position"=w677) -> ()  [unwired: 2 in, 2 out]
          n309 = property on="XY Scale Graph" class="WFGraph (strict)"("Position"=w688) -> ()  [unwired: 2 in, 2 out]
        }
      }
    }
    frame Enabled {
      # "Enable this empty diagram"
    }
  }
